vi "Unpack for gRPC.vi"(8 "error in":errorcluster, 9 "configuration / results":enum16{"Configuration", "Results"}(ring), 10 "any":T1, 11 "measurement customizations in":refnum<class "Measurement Plugin.lvclass">) -> (0 "error out":errorcluster, 2 "data value":variant, 3 "measurement customizations out":refnum<class "Measurement Plugin.lvclass">)   [LabVIEW 2021, in "Measurement Plugin.lvclass"]
uses:
  Measurement Plugin.lvclass
  <vilib>/gRPC/LabVIEW gRPC Library/Shared/Any.ctl
  C:/Program Files/National Instruments/LabVIEW 2021/vi.lib/MeasurementLink/MeasurementLink Measurement Server/Measurement Plugin Service/Measurement Plugin Service.lvclass
  Measurement Configuration.ctl
  Measurement Results.ctl
  a521b266-ce99-437c-923d-067dcf1e07fd.vi
  3ecd018e-d556-4cbc-bc60-c4ba57204520.vi
  <vilib>/gRPC/LabVIEW gRPC Library/Server API/Translate Protobuf Error.vi
  <vilib>/AdvancedString/1D String Array to Delimited String.vi
  <vilib>/gRPC/LabVIEW gRPC Library/Server API/Server/Get Server DLL Path.vi
  Measurement Plugin.lvclass/Measurement Plugin.ctl
  Stepped Frequency Sweep_Audio DAC.lvlib
  <vilib>/MeasurementLink/MeasurementLink Measurement Server/Measurement Plugin Service/Measurement Plugin Service.lvclass
  <vilib>/gRPC/LabVIEW gRPC Library/grpc-lvsupport-release.lvlib
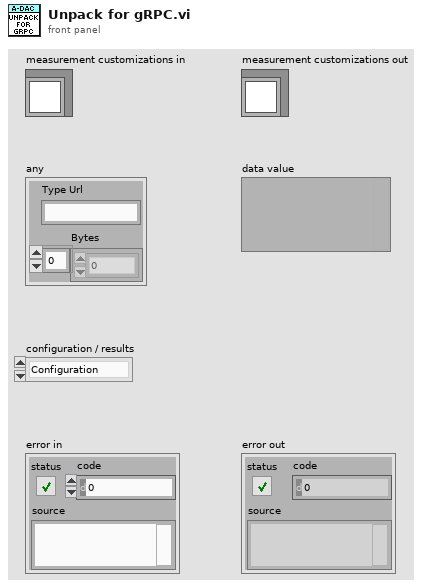
[diagram p1: front panel]
types:
  T1 = typedef "grpc-lvsupport-release.lvlib/Any.ctl" = cluster{"Type Url":string, "Bytes":u8[]}
  T2 = typedef "grpc-lvsupport-release.lvlib/grpcId.ctl" = u64
  T3 = typedef "Stepped Frequency Sweep_Audio DAC.lvlib/Measurement Configuration.ctl" = cluster{"Protocol file":string, "Digital audio channel":string, "Master clock channel":string, "Sweep Start (Hz)":dbl, "Sweep Stop (Hz)":dbl, "Sweep Steps":u32, "Sweep Profile":string, "Output level":dbl, "Output level units":string, "Output range (Vpk-pk)":dbl, "Acquisition channel":string, "Sample rate (Hz)":dbl, "Min measurement cycles":u32, "Min measurement time (s)":dbl, "Min settling cycles":u32, "Min settling time (s)":dbl, "Band start (Hz)":dbl, "Band stop (Hz)":dbl, "SNR units":string, "THD+N units":string, "THD units":string, "Gain units":string, "Highpass filter":string, "Lowpass filter":string, "Weighting filter":string}
  T4 = typedef "Stepped Frequency Sweep_Audio DAC.lvlib/Measurement Results.ctl" = cluster{"Channel names":string[], "Time domain":dbl[], "Frequency domain":dbl[], "dt":dbl, "f0":dbl, "df":dbl, "Frequency (Hz)":dbl[], "Amplitude (V)":dbl[], "Amplitude (dB)":dbl[], "Phase (deg)":dbl[], "SNR":dbl[], "THD+N":dbl[], "THD":dbl[], "Dynamic range (dB)":dbl[], "Gain":dbl[], "SFDR (dBc)":dbl[]}
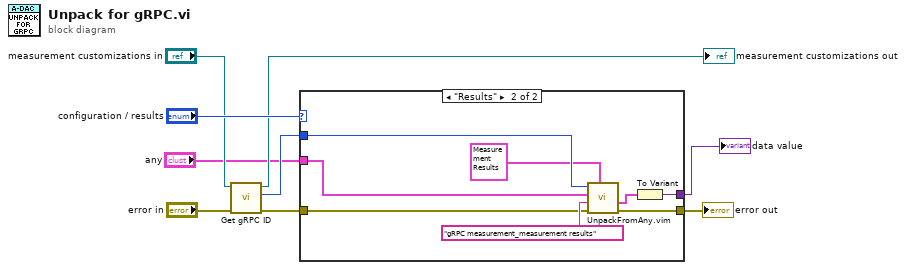
[diagram p0: block diagram]
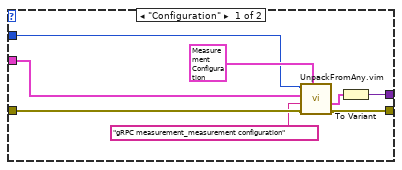
[diagram p2: hidden frame]
diagram:
  n1 = call <vilib>:"Get gRPC ID.vi"("error in"="error in", "measurement plugin service in"="measurement customizations in") -> ("error out"=w6:errorcluster, "gRPC ID"=w3:T2, "measurement plugin service out"=→"measurement customizations out":refnum<class "Measurement Plugin.lvclass">)  [unwired: 7 in]
  n2 = case shown="\"Results\"" "configuration / results" {
    tunnel: w6 -> [w15 w19]
    tunnel: "any" -> [w10 w18]
    tunnel: w3 -> [w12 w22]
    tunnel: [w16 w23] -> w9
    tunnel: [w17 w25] -> w1
    frame "Configuration" {
      n3 = call "UnpackFromAny.vim"("Data Type"=T3 {"Protocol file"="", "Digital audio channel"="", "Master clock channel"="", "Sweep Start (Hz)"=1000.0, "Sweep Stop (Hz)"=20000.0, "Sweep Steps"=11, "Sweep Profile"="Logarithmic", "Output level"=-1.0, "Output level units"="dBFS", "Output range (Vpk-pk)"=15.0, "Acquisition channel"="", "Sample rate (Hz)"=51200.0, "Min measurement cycles"=0, "Min measurement time (s)"=0.1, "Min settling cycles"=0, "Min settling time (s)"=0.1, "Band start (Hz)"=20.0, "Band stop (Hz)"=20000.0, "SNR units"="dB", "THD+N units"="dB", "THD units"="dB", "Gain units"="dB", "Highpass filter"="DC", "Lowpass filter"="No filter", "Weighting filter"="A-weighting"} ("Measurement Configuration"), "error in"=w15, "Message Type"="gRPC measurement_measurement configuration", "Any"=w10, "gRPCid in"=w12) -> ("error out"=w16:errorcluster, "Unpacked Value"=w14:T3)  [unwired: 4 in, 1 out]
      n4 = To Variant(anything=w14) -> (Variant=w17:variant)
    }
    frame "Results" {
      n5 = call "UnpackFromAny.vim"("Data Type"=T4 {"Channel names"=[], "Time domain"=[], "Frequency domain"=[], "dt"=0.0, "f0"=0.0, "df"=0.0, "Frequency (Hz)"=[], "Amplitude (V)"=[], "Amplitude (dB)"=[], "Phase (deg)"=[], "SNR"=[], "THD+N"=[], "THD"=[], "Dynamic range (dB)"=[], "Gain"=[], "SFDR (dBc)"=[]} ("Measurement Results"), "error in"=w19, "Message Type"="gRPC measurement_measurement results", "Any"=w18, "gRPCid in"=w22) -> ("error out"=w23:errorcluster, "Unpacked Value"=w24:T4)  [unwired: 4 in, 1 out]
      n6 = To Variant(anything=w24) -> (Variant=w25:variant)
    }
  }
  "error out" <- w9
  "data value" <- w1
